vi "Inficon - Set evaporator parameters.vi"(8 "Error In":errorcluster, 10 "Material refnum":refnum<vi>, 11 "COM in":refnum<visa-resource-name>) -> (0 "Error Out":errorcluster, 3 "COM out":refnum<visa-resource-name>)   [LabVIEW 2014]
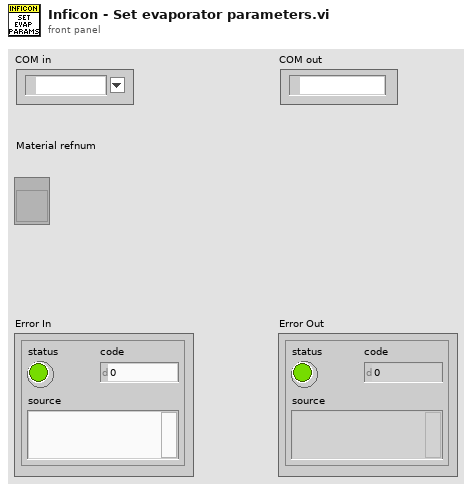
[diagram p1: front panel]
types:
  T1 = typedef "Inficon - Evaporator parameters.ctl" = cluster{"Rise Time 1 [mm:ss]":dbl, "Soak Power 1 [%]":dbl, "Soak Time 1 [mm:ss]":dbl, "Rise Time 2 [mm:ss]":dbl, "Soak Power 2 [%]":dbl, "Soak Time 2 [mm:ss]":dbl, "Shutter Delay":enum16{"No", "Yes"}, "New Rate":dbl, "Rate Ramp Time [mm:ss]":dbl, "Idle Ramp [mm:ss]":dbl, "Idle Power [%]":dbl, "Time Power":enum16{"No", "Yes"}, "Xtal Switch S":u8, "Xtal Switch Q":u8, "Tool Factor 1":dbl, "Tool Factor 2":dbl, "Deposition Rate [Å/s]":dbl, "Final Thickness [kÅ]":dbl, "Thickness Spt [kÅ]":dbl, "Density [g/cm3]":dbl, "Z-Ratio":dbl, "Sensor":u8, "Source":u8, "Crucible":u8, "Control Gain [%]":dbl, "Control TC [s]":dbl, "Control DT [s] 2":dbl, "Max Power":dbl, "Sample":u8, "Hold Time [mm:ss]":dbl}
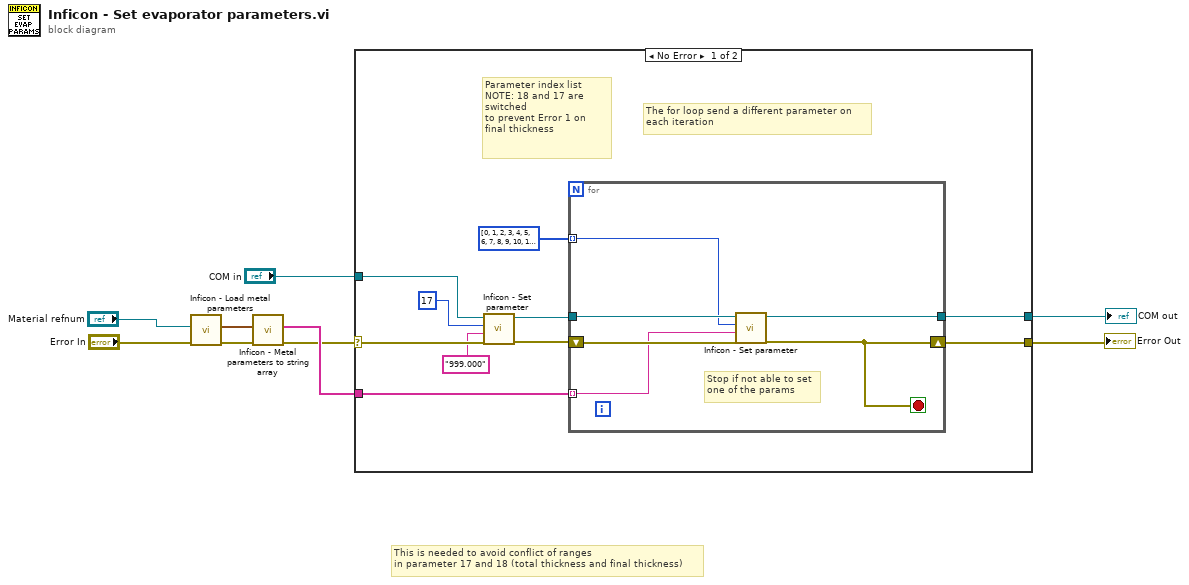
[diagram p0: block diagram]
diagram:
  # "This is needed to avoid conflict of ranges\nin parameter 17 and 18 (total thickness and final thickness)"
  n1 = call "Inficon - Load metal parameters.vi"("Error In"="Error In", "Material refnum"="Material refnum") -> ("Error Out"=w5:errorcluster, "Evaporator parameters"=w6:T1)  [unwired: 8 in]
  n2 = call "Inficon - Metal parameters to string array.vi"("Error In"=w5, "Evaporator parameters"=w6) -> ("Error Out"=w2:errorcluster, "Metal param array"=w4:string[])  [unwired: 8 in]
  n3 = case shown="No Error" w2 {
    selector: w2 -> [w13 w27]
    tunnel: [w19 w27] -> w9
    tunnel: "COM in" -> [w14 w26]
    tunnel: [w18 w26] -> w7
    tunnel: w4 -> [w17 _]
    frame No Error {
      # "Parameter index list\nNOTE: 18 and 17 are switched\nto prevent Error 1 on final thickness"
      # "The for loop send a different parameter on\neach iteration"
      n4 = call "Inficon - Set parameter.vi"("Error In"=w13, "Param value"="999.000", "Param number"=u8 17, "COM in"=w14) -> ("Error Out"=w12:errorcluster, "COM out"=w15:refnum<visa-resource-name>)  [unwired: 6 in]
      n5 = for {
        tunnel: w15 -> [w24]
        shift-right: [w22] -> w19
        shift-left: w12 -> [w25]
        tunnel: [w23] -> w18
        tunnel: w17 -> [w21] mode=indexing
        tunnel: u8[] [0, 1, 2, 3, 4, 5, 6, 7, 8, 9, 10, 11, 12, 13, 14, 15, 16, 18, 17, 19, 20, 21, 22, 23, 24, 25, 26, 27, 28, 29] -> [w20] mode=indexing
        stop <- w22 stop-if-true
        # "Stop if not able to set\none of the params"
        n6 = call "Inficon - Set parameter.vi"("Error In"=w25, "Param value"=w21, "Param number"=w20, "COM in"=w24) -> ("Error Out"=w22:errorcluster, "COM out"=w23:refnum<visa-resource-name>)  [unwired: 6 in]
      }
    }
    frame Error {
    }
  }
  "COM out" <- w7
  "Error Out" <- w9
